vi "InitProfileCurrent.vi"(8 "error in (no error)":errorcluster, 11 "StepMotor in":refnum<class "StepMotor.lvclass">) -> (0 "error out":errorcluster, 3 "StepMotor out":refnum<class "StepMotor.lvclass">)   [LabVIEW 2010, in "StepMotor.lvclass"]
uses:
  StepMotor.lvclass
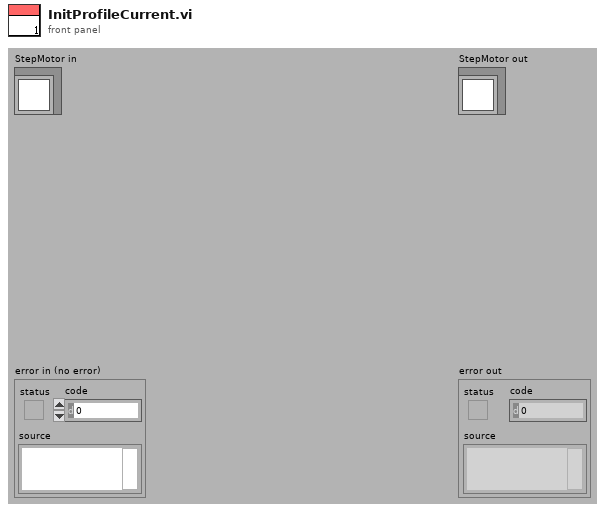
[diagram p1: front panel]
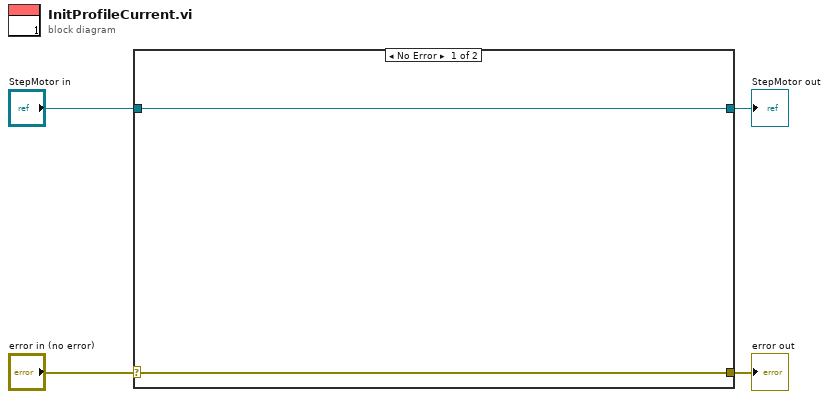
[diagram p0: block diagram]
diagram:
  n1 = case shown="No Error" "error in (no error)" {
    selector: "error in (no error)" -> [w5 w8]
    tunnel: [w5 w8] -> w3
    tunnel: [w6 w7] -> w1
    tunnel: "StepMotor in" -> [w6 w7]
    frame No Error {
    }
    frame Error {
    }
  }
  "error out" <- w3
  "StepMotor out" <- w1
